vi "Combine.vi"() -> ()   [LabVIEW 2013]
uses:
  Tools/seqs_files.ctl
  Tools/Line.ctl
panel:
  in  "Shuffle":bool
  in  "Tab Control":enum32{"Settings", "Output"}(tab)
  in  "Sequencer Files":T1=[{"Sequence File"=path "", "Repeats"=1, "Lines"=0}] caption="Input SEQs (*.osq)" {"Repeats" min=1}
  out "Lines":i32
  out "Repeats":i32
  out "Files":i32
  out "Lines":string[](array[string])
  in  "Output SEQ (*.osq)":path
  out "SEQ":T2[](array[typedef])
  in  "Stop Button":bool
  in  "Save Button":bool
  in  "Load Button":bool
  in  "Build Button":bool
  # "Combine SEQs"
  # "Total:"
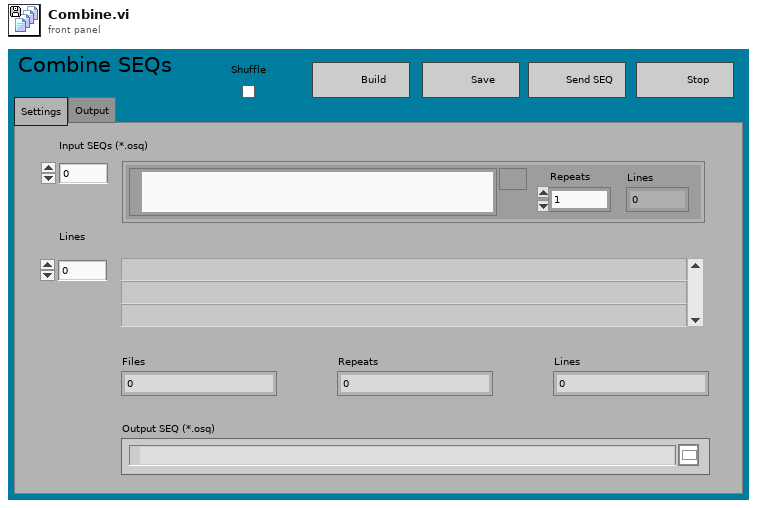
[diagram p1: front panel]
types:
  T1 = typedef "seqs_files.ctl" = cluster{"Sequence File":path, "Repeats":i32, "Lines":i32}[]
  T2 = typedef "Line.ctl" = cluster{"Var Array":string[][], "Comment":string}
  T3 = enum16{"Left Button", "Center Button", "Right Button", "Window Close"}
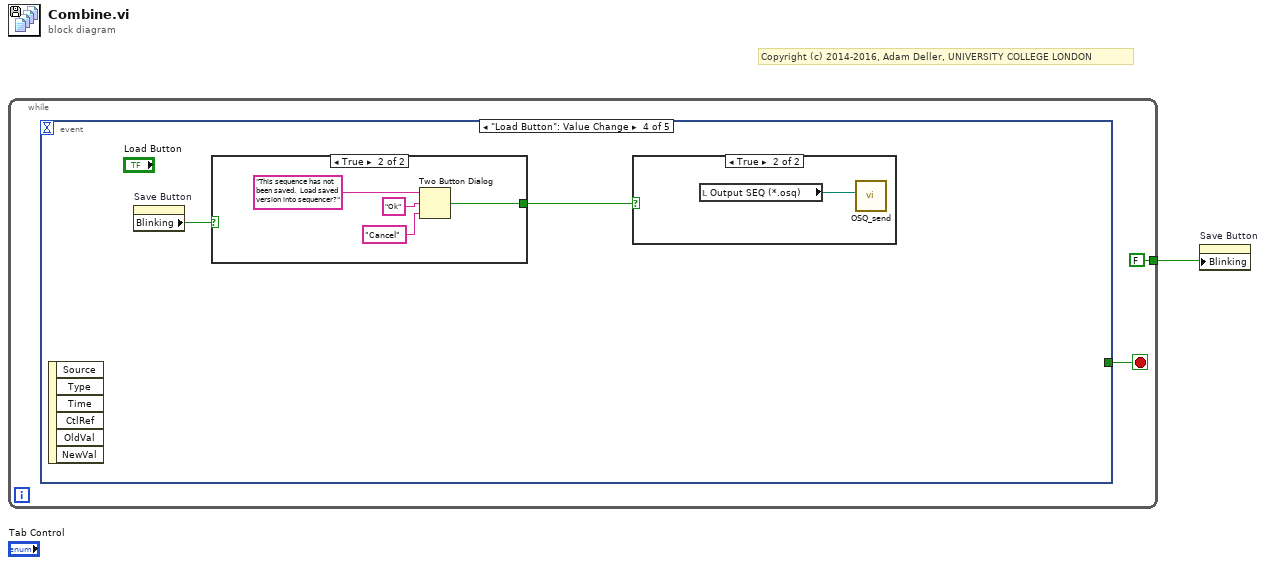
[diagram p0: block diagram]
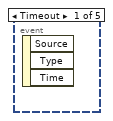
[diagram p2: hidden frame]
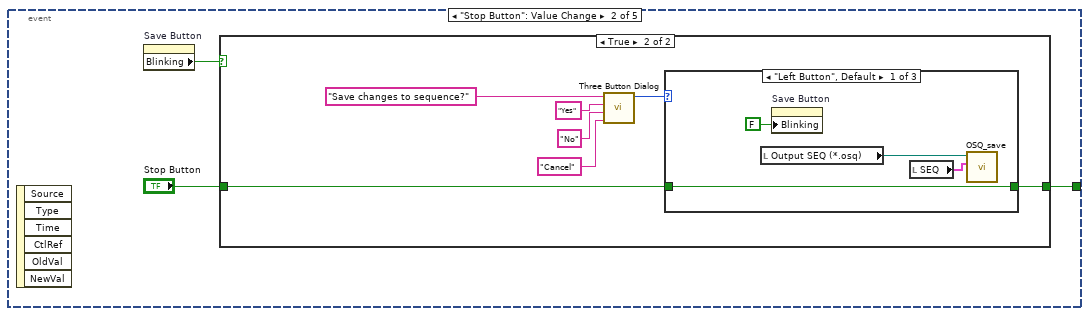
[diagram p3: hidden frame]
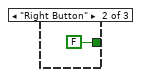
[diagram p5: hidden frame]
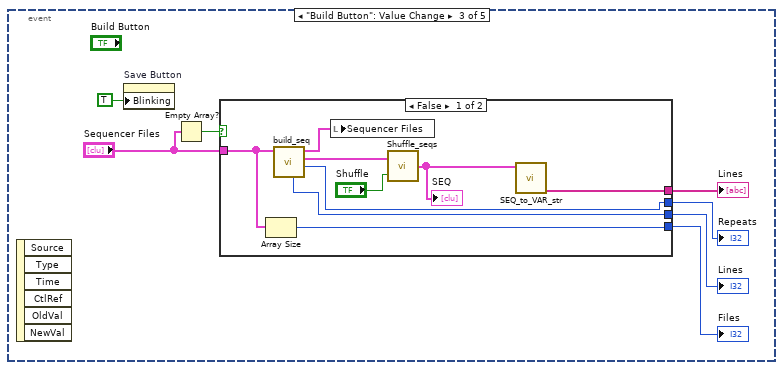
[diagram p7: hidden frame]
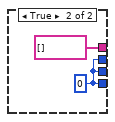
[diagram p8: hidden frame]
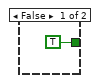
[diagram p10: hidden frame]
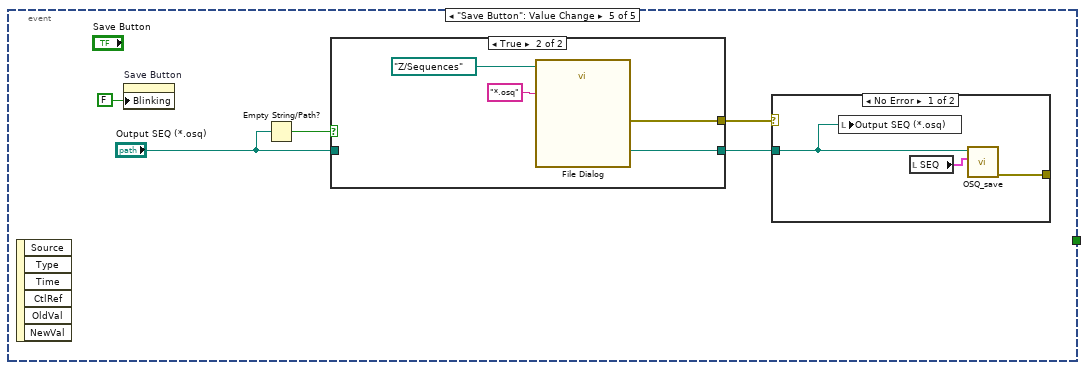
[diagram p11: hidden frame]
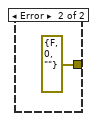
[diagram p12: hidden frame]
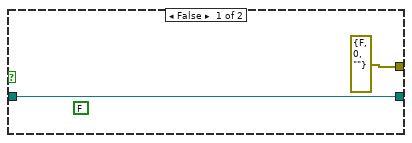
[diagram p13: hidden frame]
diagram:
  # "Copyright (c) 2014-2016, Adam Deller, UNIVERSITY COLLEGE LONDON"
  n1 = while {
    tunnel: [FALSE ("Blinking")] -> w1
    stop <- w3 stop-if-true
    n2 = event shown="[3] \"Load Button\": Value Change" {
      selector: _ -> [_ _ _ _ _]
      dyn-events: _ -> [_ _ _ _ _]
      timeout: _ -> [_ _ _ _ _]
      tunnel: [_ w4 _ _ _] -> w3
      event Timeout {
        n3 = event-data() -> ()  [unwired: 1 in, 3 out]
      }
      event "Stop Button": Value Change {
        n4 = event-data() -> ()  [unwired: 1 in, 6 out]
        n5 = property on="Save Button" class="Bool"() -> ("Blinking"=w6:bool)  [unwired: 2 in, 2 out]
        n6 = case shown="True" w6 {
          tunnel: [w7 w8] -> w4
          tunnel: "Stop Button" -> [w7 w9]
          frame False {
          }
          frame True {
            n7 = call <vilib>:"Three Button Dialog.vi"("Right Button Text (\"Cancel\")"="Cancel" ("Right Button Text (\"Cancel\")"), "Center Button Text (\"No\")"="No" ("F button name (\"Cancel\")"), "Left Button Text (\"Yes\")"="Yes" ("T button name (\"OK\")"), "message"="Save changes to sequence?") -> ("Which Button?"=w10:T3)  [unwired: 7 in]
            n8 = case shown="\"Left Button\", Default" w10 {
              tunnel: w9 -> [w18 _ w20]
              tunnel: [w18 FALSE ("Stop Button") w20] -> w8
              frame "Left Button", Default {
                n9 = local read "Output SEQ (*.osq)"() -> (w17:path)
                n10 = property on="Save Button" class="Bool"("Blinking"=FALSE) -> ()  [unwired: 2 in, 2 out]
                n11 = local read "SEQ"() -> (w15:T2[])
                n12 = call "OSQ_save.vi"("SEQs"=w15, "Save"=w17) -> ()  [unwired: 8 in, 2 out]
              }
              frame "Right Button" {
              }
              frame "Center Button" {
              }
            }
          }
        }
      }
      event "Build Button": Value Change {
        n13 = event-data() -> ()  [unwired: 1 in, 6 out]
        n14 = property on="Save Button" class="Bool"("Blinking"=TRUE) -> ()  [unwired: 2 in, 2 out]
        n15 = Empty Array?(array="Sequencer Files") -> (empty?=w22:bool)
        n16 = case shown="False" w22 {
          tunnel: "Sequencer Files" -> [w33 _]
          tunnel: [w31 string[] [] ("VAR string")] -> w23
          tunnel: [w35 w37] -> w24
          tunnel: [w34 w37] -> w25
          tunnel: [w32 w37] -> w26
          frame False {
            n17 = Array Size(array=w33) -> (size(s)=w32:i32)
            n18 = call "build_seq.vi"("Sequencer Files"=w33) -> ("Total Repeats"=w35:i32, "SEQ"=w30:T2[], "Sequence Files"=w36:T1, "Total Lines"=w34:i32)  [unwired: 5 in, 2 out]
            n19 = local write "Sequencer Files"(w36) -> ()
            n20 = call "Shuffle_seqs.vi"("Shuffle"="Shuffle", "Array IN"=w30) -> ("Array OUT"=w29:T2[])
            "SEQ" <- w29
            n21 = call "SEQ_to_VAR_str.vi"("SEQs IN"=w29) -> ("VAR Strings"=w31:string[])  [unwired: 9 in, 1 out]
          }
          frame True {
            w37 = 0 ("Total Lines")
          }
        }
        "Lines" <- w25
        "Repeats" <- w24
        "Files" <- w26
        "Lines" <- w23
      }
      event "Load Button": Value Change {
        n22 = event-data() -> ()  [unwired: 1 in, 6 out]
        n23 = property on="Save Button" class="Bool"() -> ("Blinking"=w40:bool)  [unwired: 2 in, 2 out]
        n24 = case shown="True" w40 {
          tunnel: [TRUE w43] -> w39
          frame False {
          }
          frame True {
            n25 = Two Button Dialog(message="This sequence has not been saved.  Load saved version into sequencer?", 1:"Cancel" ("F button name (\"Cancel\")"), 2:"Ok" ("T button name (\"OK\")")) -> (T button?=w43:bool)
          }
        }
        n26 = case shown="True" w39 {
          frame False {
          }
          frame True {
            n27 = local read "Output SEQ (*.osq)"() -> (w41:path)
            n28 = call "OSQ_send.vi"("Sequence File"=w41) -> ()  [unwired: 11 in]
          }
        }
      }
      event "Save Button": Value Change {
        n29 = event-data() -> ()  [unwired: 1 in, 6 out]
        n30 = property on="Save Button" class="Bool"("Blinking"=FALSE) -> ()  [unwired: 2 in, 2 out]
        n31 = Empty String/Path?(string/path="Output SEQ (*.osq)") -> (empty?=w50:bool)
        n32 = case shown="True" w50 {
          tunnel: [w57 w61] -> w49
          tunnel: "Output SEQ (*.osq)" -> [w57 _]
          tunnel: [errorcluster {"status"=FALSE, "code"=0, "source"=""} ("error out") w58] -> w48
          frame False {
            (unwired) FALSE ("cancelled")
          }
          frame True {
            n33 = call "File Dialog"("start path"=path "Z:/Sequences", "pattern (all files)"="*.osq") -> ("selected path"=w61:path, "error out"=w58:errorcluster)  [unwired: 10 in, 2 out]
          }
        }
        n34 = case shown="No Error" w48 {
          tunnel: w49 -> [w54 _]
          tunnel: [w53 errorcluster {"status"=FALSE, "code"=0, "source"=""} ("error out")] -> _
          frame No Error {
            n35 = local write "Output SEQ (*.osq)"(w54) -> ()
            n36 = local read "SEQ"() -> (w52:T2[])
            n37 = call "OSQ_save.vi"("SEQs"=w52, "Save"=w54) -> ("error out"=w53:errorcluster)  [unwired: 8 in, 1 out]
          }
          frame Error {
          }
        }
      }
    }
  }
  n38 = property on="Save Button" class="Bool"("Blinking"=w1) -> ()  [unwired: 2 in, 2 out]
